vi "Name or array position to text.vi"(7 "Array Positions (none)":i32[](array[numeric]), 10 "Name in":string) -> (2 "Name out":string)   [LabVIEW 2016, in "DCM System Explorer.lvlib"]
uses:
  DCM System Explorer.lvlib
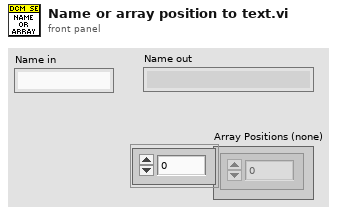
[diagram p1: front panel]
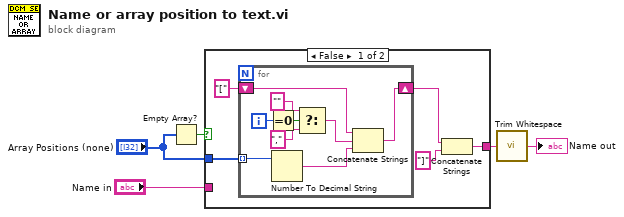
[diagram p0: block diagram]
diagram:
  n1 = Empty Array?(array="Array Positions (none)") -> (empty?=w5:bool)
  n2 = case shown="False" w5 {
    tunnel: "Array Positions (none)" -> [w10 _]
    tunnel: [w7 w20] -> w1
    tunnel: "Name in" -> [_ w20]
    frame False {
      n3 = for {
        tunnel: w10 -> [w19] mode=indexing
        shift-right: [w18] -> w8
        shift-left: "[" -> [w16]
        i -> [w11]
        n4 = Equal To 0?(x=w11) -> (x = 0?=w13:bool)
        n5 = Number To Decimal String(number=w19) -> (decimal integer string=w17:string)  [unwired: 1 in]
        n6 = Select(t="" ("string"), s=w13, f="," ("string")) -> (s? t:f=w12:string)
        n7 = Concatenate Strings(w16, w12, w17) -> (w18:string)
      }
      n8 = Concatenate Strings(w8, "]" ("string")) -> (w7:string)
    }
    frame True {
    }
  }
  n9 = call <vilib>:"Trim Whitespace.vi"("string"=w1) -> ("trimmed string"=→"Name out":string)  [unwired: 1 in]
